vi "PressureSecurityCtl.vi"(6 "FS-2 [l]":dbl, 9 "Tank Füllstandsüberwachung":bool, 10 "Füllstandsregulierung":bool, 11 "Überdruckregelung":bool) -> (3 "Füllstandsregulierung":bool)   [LabVIEW 2011]
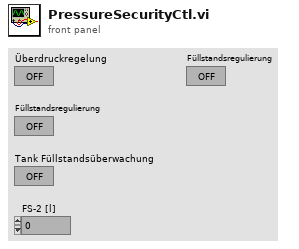
[diagram p1: front panel]
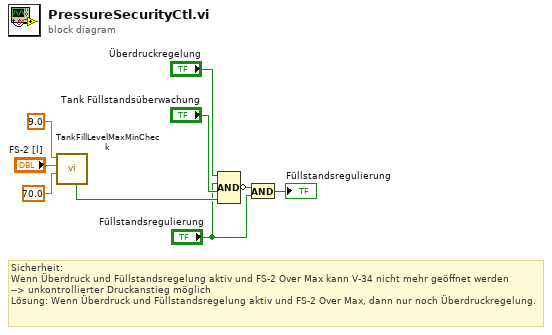
[diagram p0: block diagram]
diagram:
  # "Sicherheit:\nWenn Überdruck und Füllstandsregelung aktiv und FS-2 Over Max kann V-34 nicht mehr geöffnet werden \n--> unkontrollierter Druckanstieg möglich\nLösung: Wenn Überdruck und Füllstandsregelung aktiv und FS-2 Over Max, dann nur noch Überdruckregelung."
  n1 = call "TankFillLevelMaxMinCheck.vi"("max level"=70.0, "fill level"="FS-2 [l]", "min level"=9.0) -> ("over max"=w7:bool)  [unwired: 5 in, 3 out]
  n2 = Compound Arithmetic op=AND("Überdruckregelung", "Füllstandsregulierung", "Tank Füllstandsüberwachung", w7) -> (invert w9:bool)
  n3 = And(x=w9, y="Füllstandsregulierung") -> (x .and. y?=→"Füllstandsregulierung":bool)
